vi "Item Is Container.vi"(11 "Type String":string) -> (3 "Container?":bool)   [LabVIEW 2018, in "LVClassByRef.lvlib"]
uses:
  <resource>/Framework/Providers/LVClassByRef/LVClassByRef.lvlib
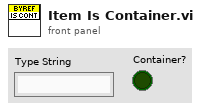
[diagram p1: front panel]
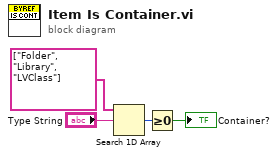
[diagram p0: block diagram]
diagram:
  n1 = Search 1D Array(1D array=string[] ["Folder", "Library", "LVClass"], element="Type String") -> (index of element=w2:i32)  [unwired: 1 in]
  n2 = Greater Or Equal To 0?(x=w2) -> (x >= 0?=→"Container?":bool)
